vi "Switch mode.vi"(2 "Galvanostatic":bool, 3 "VISA Refnum in":refnum<visa-resource-name>) -> (1 "VISA Refnum out":refnum<visa-resource-name>)   [LabVIEW 2015]
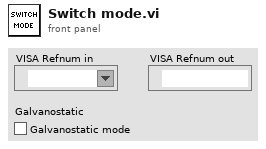
[diagram p1: front panel]
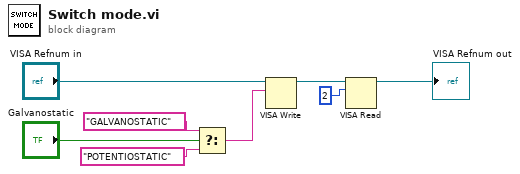
[diagram p0: block diagram]
diagram:
  n1 = Select(t="GALVANOSTATIC", s="Galvanostatic", f="POTENTIOSTATIC") -> (s? t:f=w4:string)
  n2 = VISA Write(VISA resource name="VISA Refnum in", write buffer=w4) -> (VISA resource name out=w3:refnum<visa-resource-name>)  [unwired: 1 in, 2 out]
  n3 = VISA Read(VISA resource name=w3, byte count=u32 2) -> (VISA resource name out=→"VISA Refnum out":refnum<visa-resource-name>)  [unwired: 1 in, 3 out]
